vi "Update Phasor Calibration Options Visibility.vi"(10 "Error In":errorcluster, 11 "Phasor Explorer Phasor Parameters Refnum in":refnum<vi>) -> (2 "Error Out":errorcluster, 3 "Phasor Explorer Phasor Parameters Refnum out":refnum<vi>)   [LabVIEW 2019]
uses:
  Phasor Explorer Phasor Parameters.ctl
  Phasor Calculation Type.ctl
  Phasor Type.ctl
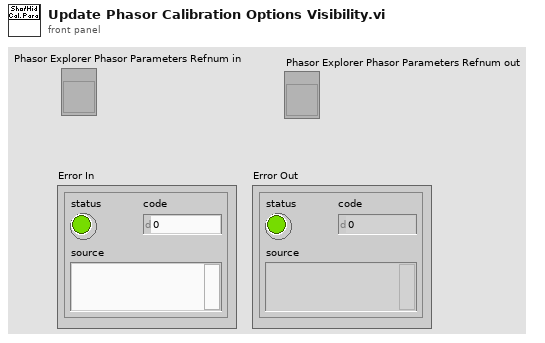
[diagram p1: front panel]
types:
  T1 = typedef "Phasor Explorer Phasor Parameters.ctl" = cluster{"Harmonic frequency":dbl[unit], "Use f* = 1/D Frequency":bool, "Calibrated Phasor":bool, "Calibration Lifetime":dbl[unit], "Phasor Calculation":T2, "SEPL Type":T3, "# Gates":dbl, "Square Gate Width":dbl[unit], "Show Ticks":bool}
  T2 = typedef "Phasor Calculation Type.ctl" = enum16{"Direct Sum", "Analytical Formula"}
  T3 = typedef "Phasor Type.ctl" = enum16{"UC", "L_N", "L_N[W]"}
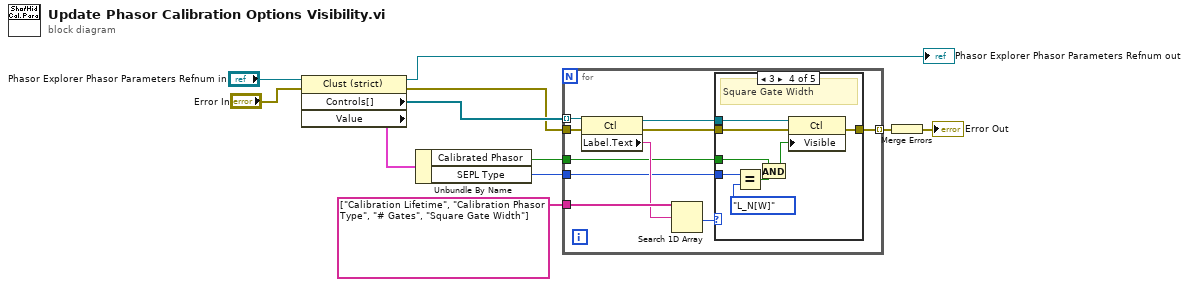
[diagram p0: block diagram]
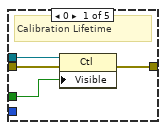
[diagram p2: hidden frame]
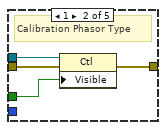
[diagram p3: hidden frame]
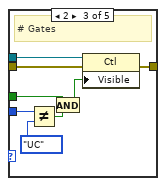
[diagram p4: hidden frame]
diagram:
  n1 = property class="Clust (strict)"(reference="Phasor Explorer Phasor Parameters Refnum in", error in="Error In") -> (reference out=→"Phasor Explorer Phasor Parameters Refnum out":refnum<vi>, error out=w5:errorcluster, "Controls[]"=w8:refnum<vi>[], "Value"=w4:T1)
  n2 = Unbundle By Name(w4) -> ("Calibrated Phasor"=w6:bool, "SEPL Type"=w1:T3)
  n3 = for {
    tunnel: w8 -> [w21] mode=indexing
    tunnel: string[] ["Calibration Lifetime", "Calibration Phasor Type", "# Gates", "Square Gate Width"] ("Label.Text") -> [w20]
    tunnel: w6 -> [w15]
    tunnel: w5 -> [w14]
    tunnel: [w13] -> w3 mode=indexing
    tunnel: w1 -> [w12]
    n4 = property class="Ctl"(reference=w21, error in=w14) -> (reference out=w17:refnum<vi>, error out=w16:errorcluster, "Label.Text"=w19:string)
    n5 = Search 1D Array(1D array=w20, element=w19) -> (index of element=w18:i32)  [unwired: 1 in]
    n6 = case shown="3" w18 {
      tunnel: w17 -> [w25 w29 w37 w45 _]
      tunnel: w16 -> [w24 w28 w36 w44 w46]
      tunnel: w15 -> [w23 w27 w30 w38 _]
      tunnel: [w22 w26 w35 w43 w46] -> w13
      tunnel: w12 -> [_ _ w34 w42 _]
      frame 0 {
        # "Calibration Lifetime"
        n7 = property class="Ctl"(reference=w25, error in=w24, "Visible"=w23) -> (error out=w22:errorcluster)  [unwired: 1 out]
      }
      frame 1 {
        # "Calibration Phasor Type"
        n8 = property class="Ctl"(reference=w29, error in=w28, "Visible"=w27) -> (error out=w26:errorcluster)  [unwired: 1 out]
      }
      frame 2 {
        # "# Gates"
        n9 = Not Equal?(x=w34, y=Phasor_Type."UC") -> (x != y?=w32:bool)
        n10 = And(x=w30, y=w32) -> (x .and. y?=w31:bool)
        n11 = property class="Ctl"(reference=w37, error in=w36, "Visible"=w31) -> (error out=w35:errorcluster)  [unwired: 1 out]
      }
      frame 3 {
        # "Square Gate Width"
        n12 = Equal?(x=w42, y=Phasor_Type."L_N[W]") -> (x = y?=w40:bool)
        n13 = And(x=w38, y=w40) -> (x .and. y?=w39:bool)
        n14 = property class="Ctl"(reference=w45, error in=w44, "Visible"=w39) -> (error out=w43:errorcluster)  [unwired: 1 out]
      }
      frame -1, Default {
      }
    }
  }
  n15 = Merge Errors(w3) -> (→"Error Out":errorcluster)
